vi "Manual_switch_EOL.vi"() -> (3 "Pass/Fail":string)   [LabVIEW 2024, in "Test_2.lvlib"]
uses:
  Test_2.lvlib
  SW_Enum_DTU.ctl
  PCANusb_DTU/support/PCAN_Global.vi
  PCANusb_DTU/PCANusb_DTU.lvlib
panel:
  in  "Instruction:":string="Press Fail only when SW1 and SW2 is not working!!!!"
  out "errorout":errorcluster
  in  "error in (no error)":errorcluster
  in  "DUT":i32
  in  "FAIL":bool
  out "DUT_S":string
  out "SW2":bool
  out "SW1":bool
  # "SWITCH FEEDBACK DUT-"
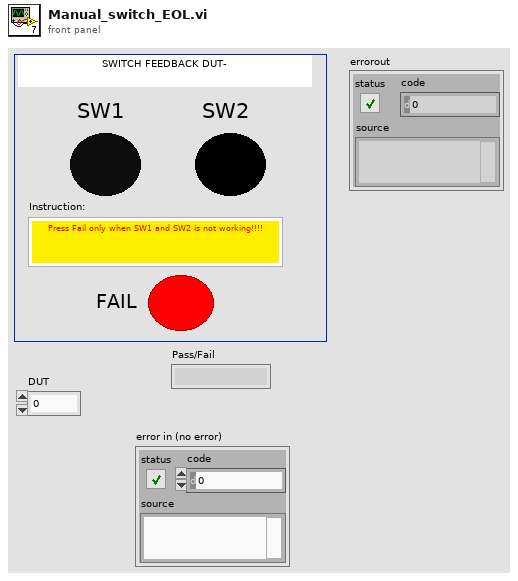
[diagram p1: front panel]
types:
  T1 = cluster{"DUT":i32, "Pass/Fail":string, "SW2":bool, "SW1":bool}
  T2 = typedef "Test_2.lvlib/SW_Enum_DTU.ctl" = enum16{"Init", "Poll", "Freeze", "Exit"}
  T3 = typedef "XNET Frame CAN.ctl" = cluster{"timestamp":timestamp, "payload":u8[], "identifier":u32, "type":T4, "extended?":bool, "echo?":bool}
  T4 = typedef "XNET Frame Type CAN.ctl" = u8
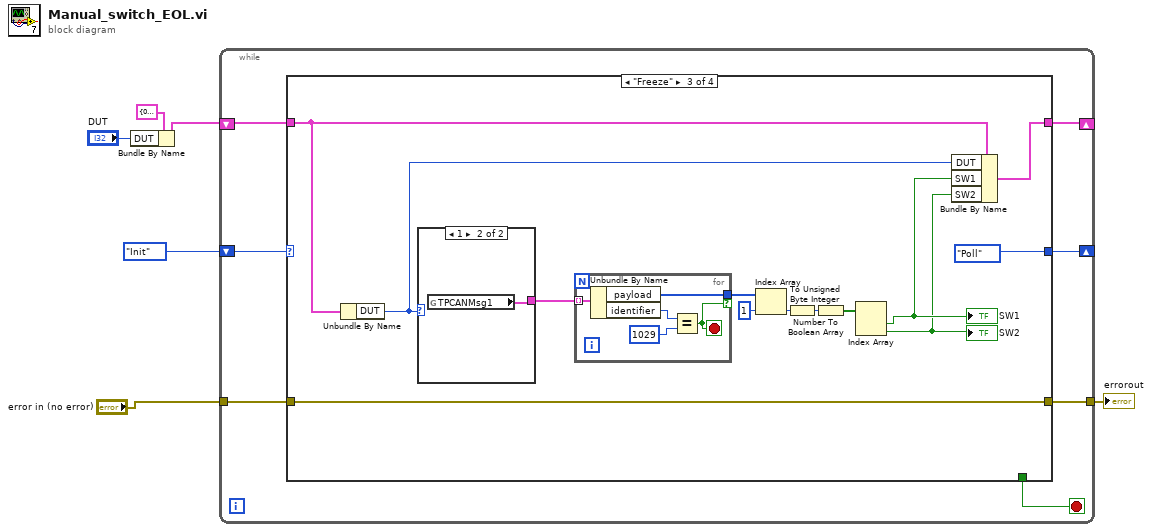
[diagram p0: block diagram]
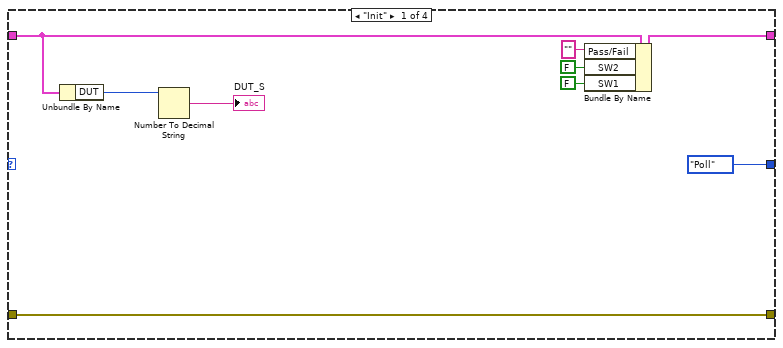
[diagram p2: hidden frame]
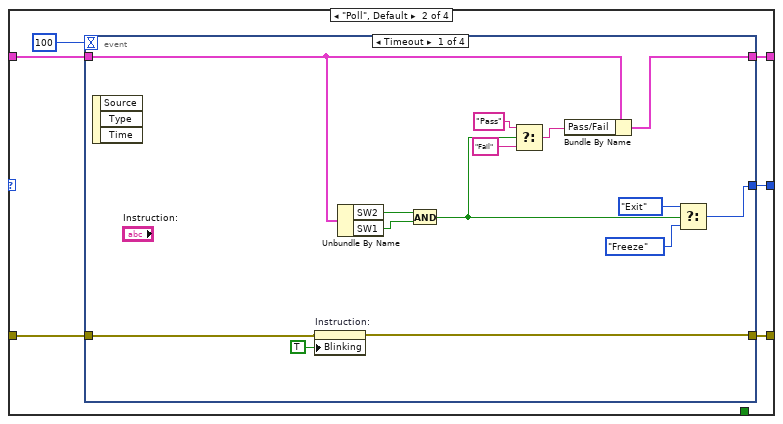
[diagram p3: hidden frame]
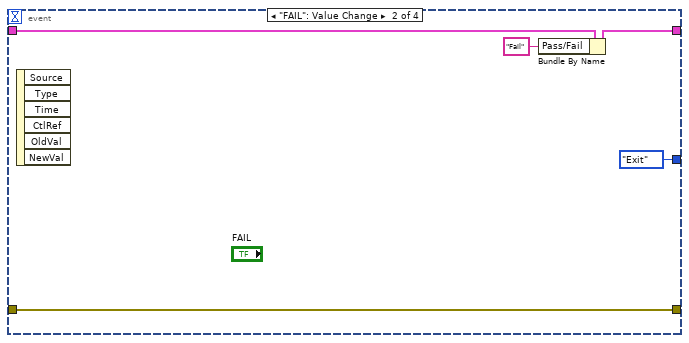
[diagram p4: hidden frame]
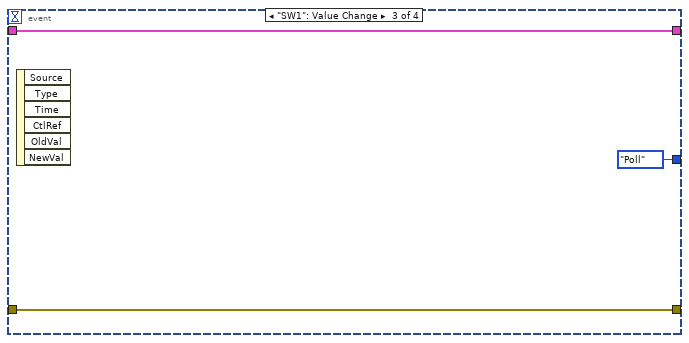
[diagram p5: hidden frame]
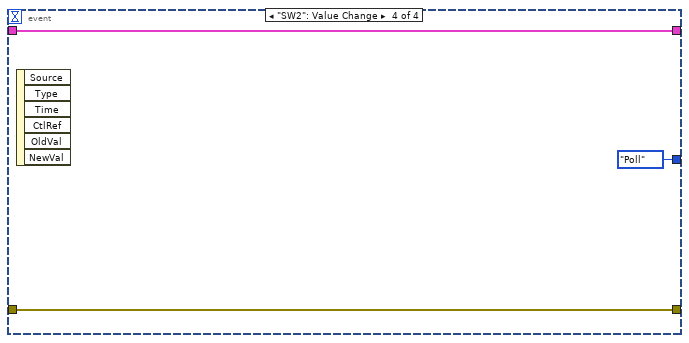
[diagram p6: hidden frame]
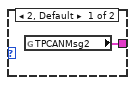
[diagram p7: hidden frame]
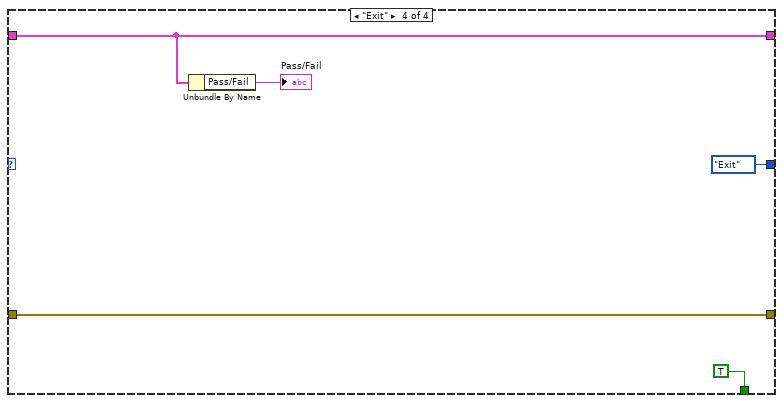
[diagram p8: hidden frame]
diagram:
  n1 = Bundle By Name(cluster=T1 {"DUT"=0, "Pass/Fail"="", "SW2"=FALSE, "SW1"=FALSE}, "DUT"="DUT") -> (w5:T1)
  n2 = while {
    shift-right: [w11] -> _
    shift-left: w5 -> [w12]
    tunnel: "error in (no error)" -> [w10]
    tunnel: [w9] -> w2
    shift-right: [w7] -> _
    shift-left: SW_Enum_DTU."Init" -> [w8]
    stop <- w13 stop-if-true
    n3 = case shown="\"Freeze\"" w8 {
      tunnel: [_ _ _ TRUE] -> w13
      tunnel: w12 -> [w22 w27 w65 w76]
      tunnel: [w19 w26 w64 w76] -> w11
      tunnel: w10 -> [w15 w24 w66 w77]
      tunnel: [w15 w25 w66 w77] -> w9
      tunnel: [SW_Enum_DTU."Poll" w23 SW_Enum_DTU."Poll" SW_Enum_DTU."Exit"] -> w7
      frame "Init" {
        n4 = Unbundle By Name(w22) -> ("DUT"=w21:i32)
        n5 = Number To Decimal String(number=w21) -> (decimal integer string=→"DUT_S":string)  [unwired: 1 in]
        n6 = Bundle By Name(cluster=w22, "Pass/Fail"="", "SW2"=FALSE, "SW1"=FALSE) -> (w19:T1)
      }
      frame "Poll", Default {
        n7 = event shown="[0] Timeout" {
          selector: _ -> [_ _ _ _]
          dyn-events: _ -> [_ _ _ _]
          timeout: 100 -> [_ _ _ _]
          tunnel: [w37 SW_Enum_DTU."Exit" SW_Enum_DTU."Poll" SW_Enum_DTU."Poll"] -> w23
          tunnel: w27 -> [w42 w46 w49 w52]
          tunnel: [w36 w44 w49 w52] -> w26
          tunnel: [w30 w45 w48 w51] -> w25
          tunnel: w24 -> [w31 w45 w48 w51]
          event Timeout {
            n8 = event-data() -> ()  [unwired: 1 in, 3 out]
            n9 = property on="Instruction:" class="Str"(error in=w31, "Blinking"=TRUE) -> (error out=w30:errorcluster)  [unwired: 1 in, 1 out]
            n10 = Unbundle By Name(w42) -> ("SW2"=w40:bool, "SW1"=w41:bool)
            n11 = And(x=w40, y=w41) -> (x .and. y?=w35:bool)
            n12 = Select(t="Pass", s=w35, f="Fail") -> (s? t:f=w32:string)
            n13 = Bundle By Name(cluster=w42, "Pass/Fail"=w32) -> (w36:T1)
            n14 = Select(t=SW_Enum_DTU."Exit", s=w35, f=SW_Enum_DTU."Freeze") -> (s? t:f=w37:T2)
          }
          event "FAIL": Value Change {
            n15 = event-data() -> ()  [unwired: 1 in, 6 out]
            n16 = Bundle By Name(cluster=w46, "Pass/Fail"="Fail") -> (w44:T1)
          }
          event "SW1": Value Change {
            n17 = event-data() -> ()  [unwired: 1 in, 6 out]
          }
          event "SW2": Value Change {
            n18 = event-data() -> ()  [unwired: 1 in, 6 out]
          }
        }
      }
      frame "Freeze" {
        n19 = Unbundle By Name(w65) -> ("DUT"=w63:i32)
        n20 = case shown="1" w63 {
          tunnel: [w72 w73] -> w54
          frame 2, Default {
            n21 = global read "PCAN_Global.vi" "TPCANMsg2"() -> (w72:T3[])
          }
          frame 1 {
            n22 = global read "PCAN_Global.vi" "TPCANMsg1"() -> (w73:T3[])
          }
        }
        n23 = for {
          tunnel: [w69] -> w59 if=w68
          tunnel: w54 -> [w67] mode=indexing
          stop <- w68 stop-if-true
          n24 = Unbundle By Name(w67) -> ("payload"=w69:u8[], "identifier"=w70:u32)
          n25 = Equal?(x=w70, y=u32 1029 ("identifier")) -> (x = y?=w68:bool)
        }
        n26 = Index Array(array=w59, index=1) -> (element=w57:u8)
        n27 = To Unsigned Byte Integer(number=w57) -> (unsigned 8bit integer=w56:u8)
        n28 = Number To Boolean Array(number=w56) -> (Boolean array=w55:bool[])
        n29 = Index Array(array=w55) -> (element #1=w62:bool, element #2=w61:bool)  [unwired: 2 in]
        "SW1" <- w62
        "SW2" <- w61
        n30 = Bundle By Name(cluster=w65, "DUT"=w63, "SW1"=w62, "SW2"=w61) -> (w64:T1)
      }
      frame "Exit" {
        n31 = Unbundle By Name(w76) -> ("Pass/Fail"=→"Pass/Fail":string)
      }
    }
  }
  "errorout" <- w2
